vi "Read Attributes.vi"(11 "Abstract Message Template in":refnum<class "Show or Hide Quick Settings Msg.lvclass">) -> (3 "Abstract Message Template out":refnum<class "Show or Hide Quick Settings Msg.lvclass">)   [LabVIEW 2014, in "HIJ Vision Display.lvlib" / "Show or Hide Quick Settings Msg.lvclass"]
uses:
  Show or Hide Quick Settings Msg.lvclass
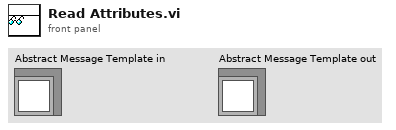
[diagram p1: front panel]
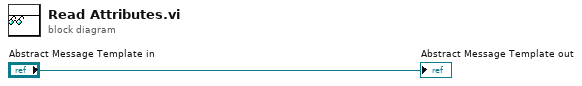
[diagram p0: block diagram]
diagram:
  "Abstract Message Template out" <- "Abstract Message Template in"
